vi "20TILM_Set_Monitor_Values.vi"(1 "20TILM Status":T1, 2 "System Monitor Variables (in)":T2) -> (0 "System Monitor Variables (out)":T2)   [LabVIEW 2019]
uses:
  Global/Global Variables/System Monitor Cluster.ctl
  Gustav/20TILM_Status.ctl
panel:
  # "Levelmeter"
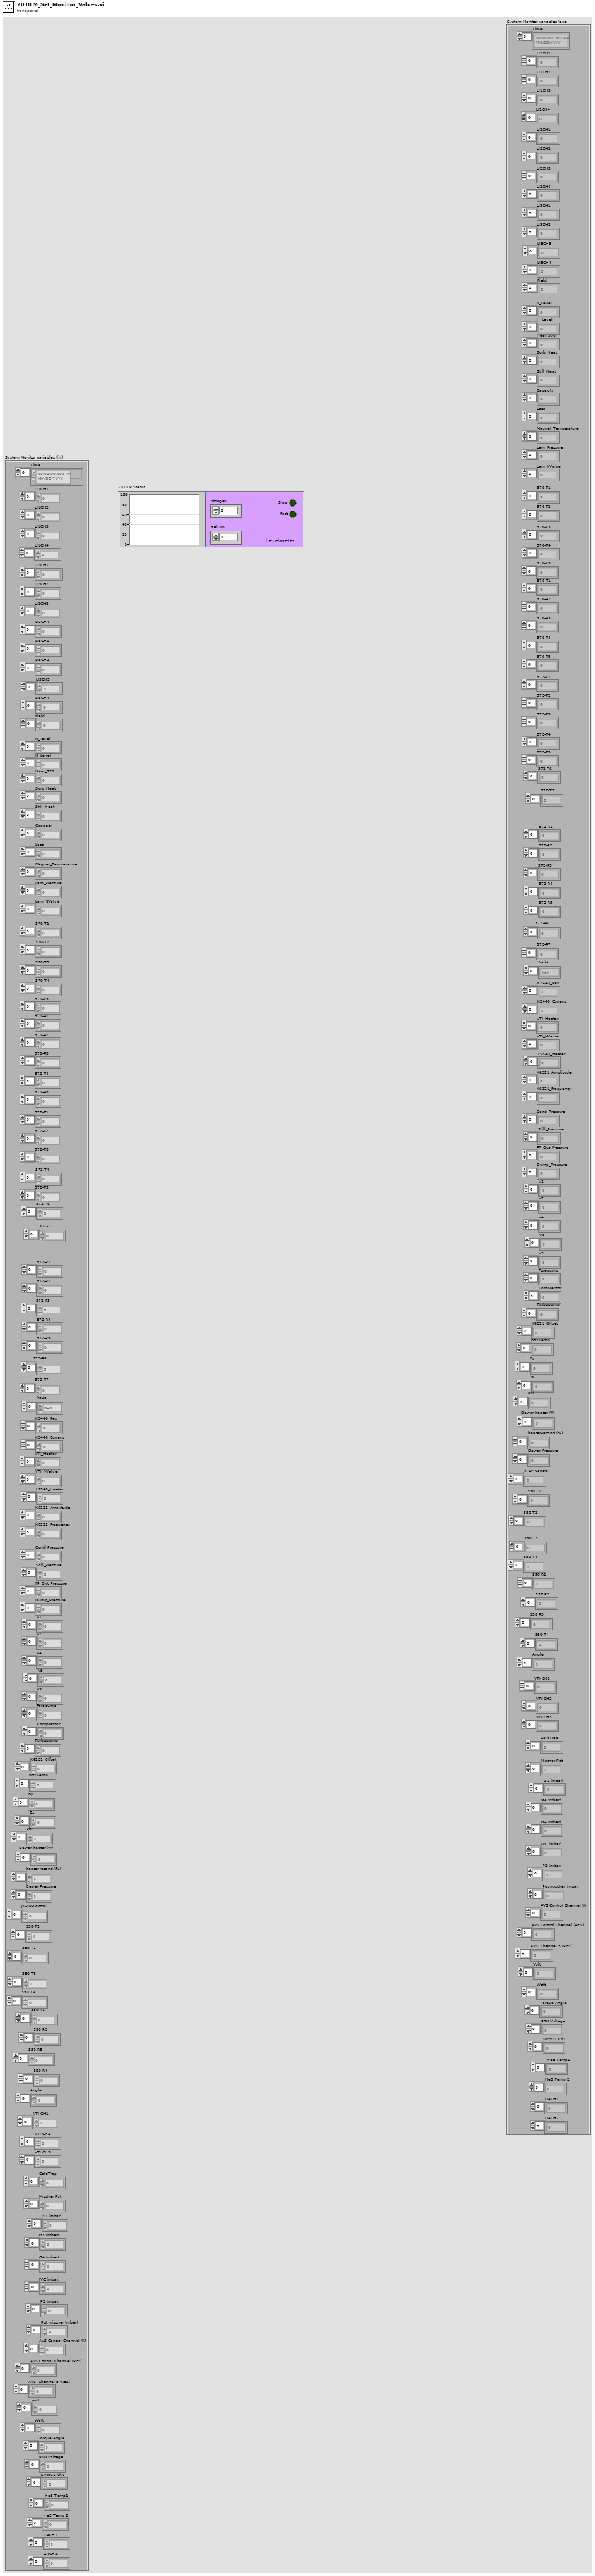
[diagram p1: front panel]
types:
  T1 = typedef "20TILM_Status.ctl" = cluster{"Helium":dbl, "Nitrogen":dbl, "Slow":bool, "Fast":bool, "Plot":cluster{"X":dbl, "Y":dbl}[]}
  T2 = typedef "System Monitor Cluster.ctl" = cluster{"Time":timestamp[], "LI1CH1":dbl[], "LI1CH2":dbl[], "LI2CH1":dbl[], "LI2CH2":dbl[], "LI3CH1":dbl[], "LI3CH2":dbl[], "Field":dbl[], "N_Level":dbl[], "H_Level":dbl[], "Heat_370":dbl[], "Sorb_Heat":dbl[], "Still_Heat":dbl[], "Capacity":dbl[], "Loss":dbl[], "Magnet_Temperature":dbl[], "Lam_Pressure":dbl[], "Lam_NValve":dbl[], "370-T1":dbl[], "370-T2":dbl[], "370-T3":dbl[], "370-T4":dbl[], "370-T5":dbl[], "370-R1":dbl[], "370-R2":dbl[], "370-R3":dbl[], "370-R4":dbl[], "370-R5":dbl[], "372-T1":dbl[], "372-T2":dbl[], "372-T3":dbl[], "372-T4":dbl[], "372-T5":dbl[], "372-T6":dbl[], "372-R1":dbl[], "372-R2":dbl[], "372-R3":dbl[], "372-R4":dbl[], "372-R5":dbl[], "372-R6":dbl[], "Nada":dbl[], "K2440_Res":dbl[], "K2440_Current":dbl[], "VTI_Heater":dbl[], "VTI_NValve":dbl[], "LS340_Heater":dbl[], "K6221_Amplitude":dbl[], "K6221_Frequency":dbl[], "Cond_Pressure":dbl[], "Still_Pressure":dbl[], "FP_Out_Pressure":dbl[], "Dump_Pressure":dbl[], "V1":dbl[], "V2":dbl[], "V4":dbl[], "V5":dbl[], "V9":dbl[], "Forepump":dbl[], "Compressor":dbl[], "K6221_Offset":dbl[], "BoxTemp":dbl[], "By":dbl[], "Bz":dbl[], "Phi":dbl[], "heater-recond (%)":dbl[], "Dewar Pressure ":dbl[], "JT-SP-Control":dbl[], "350 T1":dbl[], "350 T2":dbl[], "350 T3":dbl[], "350 T4":dbl[], "350 R1":dbl[], "350 R2":dbl[], "350 R3":dbl[], "350 R4":dbl[], "Angle":dbl[], "VTI CH1":dbl[], "VTI CH2":dbl[], "VTI CH3":dbl[], "ColdTrap":dbl[], "Mischer Pot":dbl[], "G1 (mbar)":dbl[], "G3 (mbar) ":dbl[], "G4 (mbar)":dbl[], "IVC (mbar)":dbl[], "P2 (mbar) ":dbl[], "Pot mischer (mbar)":dbl[], "AVS Control Channel (K)":dbl[], "AVS Control Channel (RES)":dbl[], "AVS  Channel 5 (RES) ":dbl[], "LI3CH3":dbl[], "LI3CH4":dbl[], "LI1CH3":dbl[], "LI1CH4":dbl[], "LI2CH3":dbl[], "LI2CH4":dbl[], "Volt":dbl[], "Watt":dbl[], "Torque Angle":dbl[], "Dewar heater (W)":dbl[], "PSU Voltage":dbl[], "Turbopump":dbl[], "372-R7":dbl[], "372-T7":dbl[], "SIM921 Ch1":dbl[], " He3 Temp1":dbl[], " He3 Temp 2":dbl[], "LI4CH1":dbl[], "LI4CH2":dbl[]}
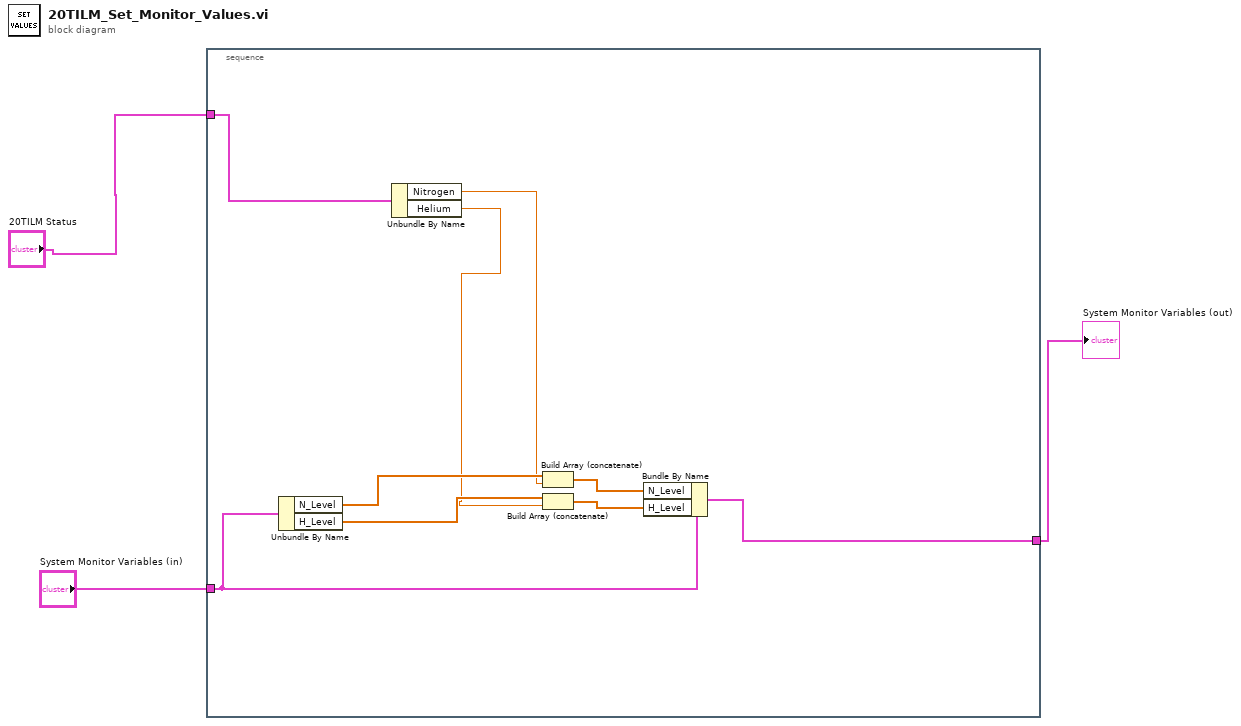
[diagram p0: block diagram]
diagram:
  n1 = stacked-sequence {
    tunnel: "System Monitor Variables (in)" -> [w5]
    tunnel: [w8] -> w2
    tunnel: "20TILM Status" -> [w4]
    frame #0 {
      n2 = Unbundle By Name(w5) -> ("N_Level"=w12:dbl[], "H_Level"=w11:dbl[])
      n3 = Unbundle By Name(w4) -> ("Nitrogen"=w10:dbl, "Helium"=w9:dbl)
      n4 = Build Array (concatenate)(w12, w10) -> (w7:dbl[])
      n5 = Build Array (concatenate)(w11, w9) -> (w6:dbl[])
      n6 = Bundle By Name(cluster=w5, "N_Level"=w7, "H_Level"=w6) -> (w8:T2)
    }
  }
  "System Monitor Variables (out)" <- w2
